vi "Read V2 Trigger Settings.vi"(8 "error in (no error)":errorcluster, 11 "BME_DG_G05 in":refnum<class "BME_DG_G05.lvclass">) -> (0 "error out":errorcluster, 2 "V2 Trigger Settings":T1, 3 "BME_DG_G05 out":refnum<class "BME_DG_G05.lvclass">)   [LabVIEW 2009, in "POLARIS BME DG.lvlib" / "BME_DG_G05.lvclass"]
uses:
  BME_DG_G05.lvclass
  BME_DG_G05.lvclass/BME_DG_G05.ctl
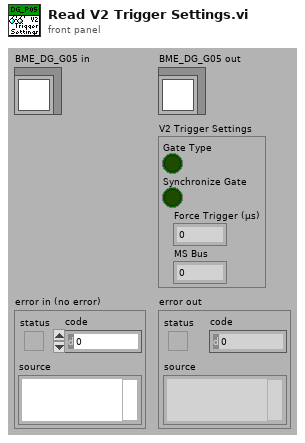
[diagram p1: front panel]
types:
  T1 = cluster{"Gate Type":bool, "Synchronize Gate":bool, "Force Trigger (µs)":dbl, "MS Bus":u32}
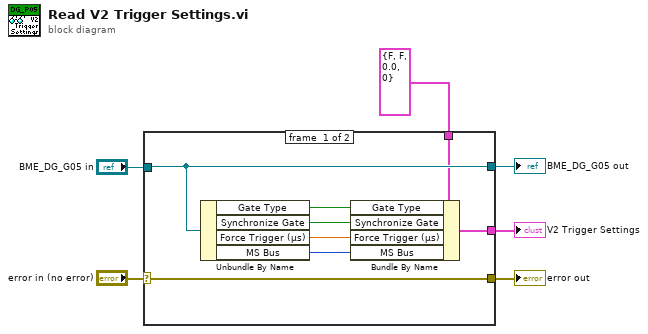
[diagram p0: block diagram]
diagram:
  n1 = case shown="No Error" "error in (no error)" {
    selector: "error in (no error)" -> [w10 w16]
    tunnel: [w9 w15] -> w6
    tunnel: "BME_DG_G05 in" -> [w9 w15]
    tunnel: [w10 w16] -> w3
    tunnel: [w8 _] -> w2
    tunnel: T1 {"Gate Type"=FALSE, "Synchronize Gate"=FALSE, "Force Trigger (µs)"=0.0, "MS Bus"=0} ("V2 Trigger Settings") -> [w7 _]
    frame #0 {
      n2 = Unbundle By Name(w9) -> ("Gate Type"=w14:bool, "Synchronize Gate"=w12:bool, "Force Trigger (µs)"=w11:dbl, "MS Bus"=w13:u32)
      n3 = Bundle By Name(cluster=w7, "Gate Type"=w14, "Synchronize Gate"=w12, "Force Trigger (µs)"=w11, "MS Bus"=w13) -> (w8:T1)
    }
    frame #1 {
    }
  }
  "error out" <- w3
  "BME_DG_G05 out" <- w6
  "V2 Trigger Settings" <- w2
